vi "Initialise.vi"(8 "error in (no error)":errorcluster, 10 "Message in":refnum<class "InitialiseMessage.lvclass">, 11 "ConfocalStage in":refnum<class "ConfocalStage.lvclass">) -> (0 "error out":errorcluster, 3 "ConfocalStage out":refnum<class "ConfocalStage.lvclass">)   [LabVIEW 2012, in "ConfocalStage.lvclass"]
doc: "This method is called when an initialise message is received. It mainly initialises the RabbitMQ connectivity. \n\nOverride this method when your component needs special initialisation (e.g. of software or hardware resources). In that case, don't forget to call the parent for proper implementation. If your component owns subcomponents, they count as resources, so you have to initialise them by calling their own initialise functions"
uses:
  ConfocalStage.lvclass
  <vilib>/Distrio/Murmex/InitialiseMessage/InitialiseMessage.lvclass
  <vilib>/Distrio/Murmex/Murmex/Murmex.lvclass
  ConfocalStage.lvclass/ConfocalStage.ctl
panel:
  # "This method is called when the INTIALISE\ntrigger is sent. \n\nOverride this method when your component needs to\nrespond to this trigger. \n\nCall parent for proper implementation"
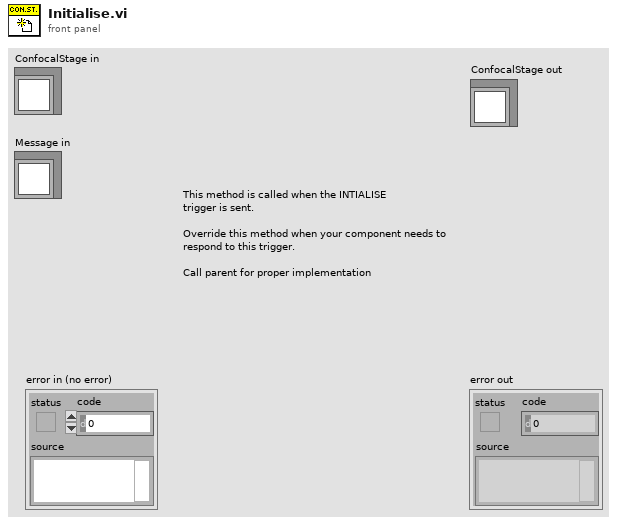
[diagram p1: front panel]
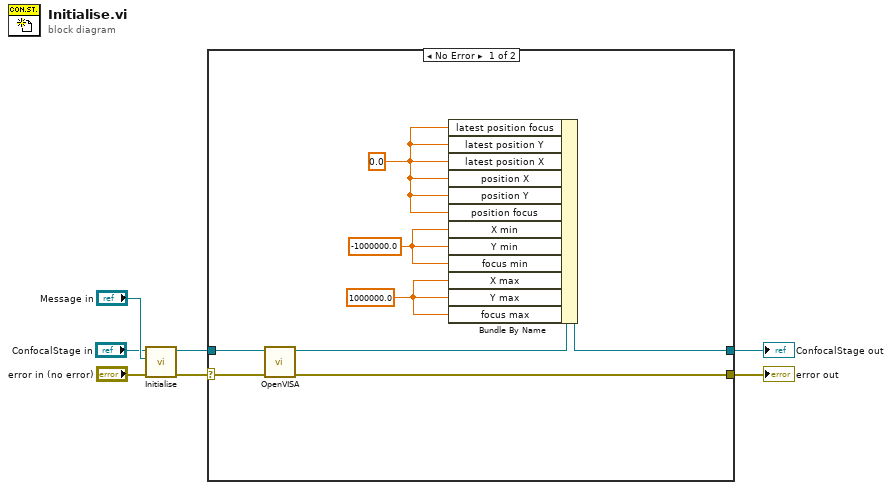
[diagram p0: block diagram]
diagram:
  n1 = call-parent "Initialise.vi"("error in (no error)"="error in (no error)", "Message in"="Message in", "Murmex in"="ConfocalStage in") -> ("error out"=w4:errorcluster, "Murmex out"=w1:refnum<class "ConfocalStage.lvclass">)  [unwired: 7 in]
  n2 = case shown="No Error" w4 {
    selector: w4 -> [w14 w17]
    tunnel: [w9 w17] -> w3
    tunnel: [w10 w16] -> w2
    tunnel: w1 -> [w15 w16]
    frame No Error {
      w11 = 1000000.0 ("runtime.X min")
      w12 = -1000000.0 ("runtime.X min")
      w8 = 0.0 ("runtime.position X")
      n3 = call-dynamic "OpenVISA.vi"("error in (no error)"=w14, "ConfocalStage in"=w15) -> ("error out"=w9:errorcluster, "ConfocalStage out"=w13:refnum<class "ConfocalStage.lvclass">)  [unwired: 8 in]
      n4 = Bundle By Name(cluster=w13, "latest position focus"=w8, "latest position Y"=w8, "latest position X"=w8, "position X"=w8, "position Y"=w8, "position focus"=w8, "X min"=w12, "Y min"=w12, "focus min"=w12, "X max"=w11, "Y max"=w11, "focus max"=w11) -> (w10:refnum<class "ConfocalStage.lvclass">)
    }
    frame Error {
    }
  }
  "error out" <- w3
  "ConfocalStage out" <- w2
